vi "RichToFlatGreeter_req.vi"(5 "OutputClusterType":T1, 11 "InputCluster":T3) -> (3 "OutputCluster":T1)   [LabVIEW 2019, in "Generated_server.lvlib"]
uses:
  Generated_server.lvlib
  Greeter_req.ctl
  Greeter_req_req_oneof/Greeter_req_req_oneof.lvclass
  Greeter_req_Flat.ctl
  Greeter_MessageA_Flat.ctl
  Greeter_req_req_oneof/Greeter_req_req_oneof.lvclass/Greeter_req_req_oneof.ctl
  Greeter_MessageA_oneof_a/Greeter_MessageA_oneof_a.lvclass/Greeter_MessageA_oneof_a.ctl
  Greeter_MessageA_oneof_a/Getdata_a1.vi
  Greeter_MessageA_oneof_a/Getdata_a2.vi
  Greeter_MessageA_oneof_a/Greeter_MessageA_oneof_a.lvclass
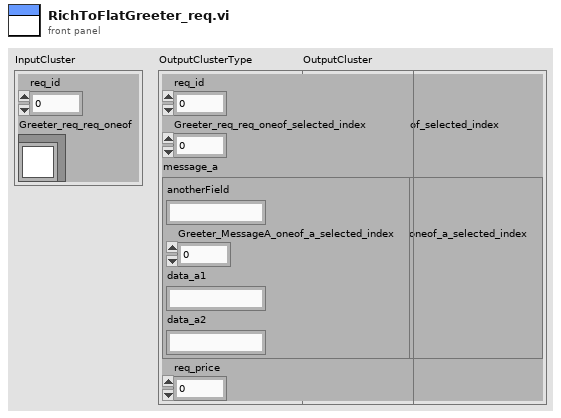
[diagram p1: front panel]
types:
  T1 = typedef "Generated_server.lvlib/Greeter_req_Flat.ctl" = cluster{"req_id":i32, "Greeter_req_req_oneof_selected_index":i32, "message_a":T2, "req_price":dbl}
  T2 = typedef "Generated_server.lvlib/Greeter_MessageA_Flat.ctl" = cluster{"anotherField":string, "Greeter_MessageA_oneof_a_selected_index":i32, "data_a1":string, "data_a2":string}
  T3 = typedef "Generated_server.lvlib/Greeter_req.ctl" = cluster{"req_id":i32, "Greeter_req_req_oneof":refnum<class "Greeter_req_req_oneof.lvclass">}
  T4 = typedef "Generated_server.lvlib/Greeter_MessageA.ctl" = cluster{"anotherField":string, "Greeter_MessageA_oneof_a":refnum<class "Greeter_MessageA_oneof_a.lvclass">}
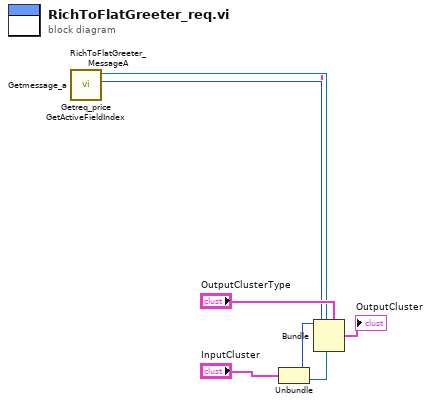
[diagram p0: block diagram]
diagram:
  n1 = Unbundle "Unbundle"("InputCluster") -> ("req_id"=w6:i32, "Greeter_req_req_oneof"=w5:refnum<class "Greeter_req_req_oneof.lvclass">)
  n2 = call "Getreq_price.vi"("OneOfTemplate in"=w5) -> ("Get_Val"=w1:dbl)  [unwired: 8 in, 2 out]
  n3 = call "Getmessage_a.vi"("OneOfTemplate in"=w5) -> ("Get_Val"=w3:T4)  [unwired: 8 in, 2 out]
  n4 = call "RichToFlatGreeter_MessageA.vi"("InputCluster"=w3) -> ("OutputCluster"=w2:T2)  [unwired: 10 in]
  n5 = call "GetActiveFieldIndex.vi"("OneOfTemplate in"=w5) -> ("Active Field Index"=w4:i32)  [unwired: 8 in, 2 out]
  n6 = Bundle "Bundle"(cluster="OutputClusterType", "req_id"=w6, "Greeter_req_req_oneof_selected_index"=w4, "message_a"=w2, "req_price"=w1) -> (→"OutputCluster":T1)
